vi "Shell and Tube Heat Exchanger 2.vi"() -> ()   [LabVIEW 2017]
uses:
  FlowSet S&THx.vi
  Level Set S&THx.vi
  Steam Set S&THx.vi
  Halt S&THx.vi
  <vilib>/addons/control/pid/pid.llb/PID Control Input Filter (DBL).vi
  <vilib>/addons/control/pid/pid.llb/PID Advanced (DBL).vi
  Flow Out S&THx.vi
  Level Out S&THx.vi
  Steam Out S&THx.vi
  <vilib>/addons/control/pid/NI_PID_pid.lvlib
panel:
  in  "Recording Increment (sec)":dbl=0.3 min=0.1 max=100.0 step=0.1 format="%#_13g"
  in  "stop":bool
  out "Last Time Write":dbl format="%#_13g"
  in  "Replace File":bool
  in  "Enable 6":bool
  in  "error in (no error)":errorcluster
  out "Makeup Flowrate":dbl caption="L/min"
  out "Makeup Temperature":dbl caption="C"
  in  "Pump Switch":bool
  out "Water Inlet Temperature":dbl=22.229346791369398 format="%.1f"
  out "Water Outlet Temperature":dbl=22.816489944987293 format="%.1f"
  in  "Flowrate Setpoint (GPM)":dbl=40.0 min=0.0 max=50.0 format="%.2f"
  out "Water Flowrate":dbl=-0.0005338564515105265 format="%.2f"
  out "Flow Control Valve":dbl(slide)=100.0 scale=0.0..100.0
  in  "Manual Override (Flow)":bool=TRUE
  in  "Set Manual Valve Position (Flow)":dbl(slide)=100.0 scale=0.0..100.0
  in  "Level Setpoint (ft)":dbl=1.5 min=0.0 max=2.0 format="%.2f"
  out "Liquid Level in Tank":dbl=-0.5117058749718749 format="%.2f"
  out "Level Control Valve":dbl(slide)=0.045055175643920364 scale=0.0..100.0
  in  "Manual Override (Level)":bool=TRUE
  in  "Set Manual Valve Position (Level)":dbl(slide) scale=0.0..100.0
  in  "Kc (Flow)":dbl=0.74
  in  "Ti (Flow)":dbl=0.036 caption="(min)"
  in  "Td (Flow)":dbl caption="(min)"
  in  "Kc (Level)":dbl=-75.0
  in  "Ti (Level)":dbl=0.005 caption="(min)"
  in  "Td (Level)":dbl caption="(min)"
  out "House Steam Pressure":dbl=-37.74410859375 caption="psig" format="%#.6g"
  out "Tube-Side Pressure Drop":dbl=-3.6907662628125 caption="psig"
  in  "Main Power":bool
  in  "Steam Pressure Setpoint (psig)":dbl=10.0 min=0.0 max=45.0 format="%.2f"
  out "Steam Pressure":dbl=-38.330115825 caption="psig" format="%.2f"
  out "Steam Valve":dbl(slide) scale=0.0..100.0
  in  "Manual Control Override (Steam Pressure)":bool
  in  "Set Manual Valve Position (Steam Pressure)":dbl(slide) scale=0.0..100.0
  in  "Kc (Steam)":dbl=0.5
  in  "Ti (Steam)":dbl=0.05 caption="(min)"
  in  "Td (Steam)":dbl caption="(min)"
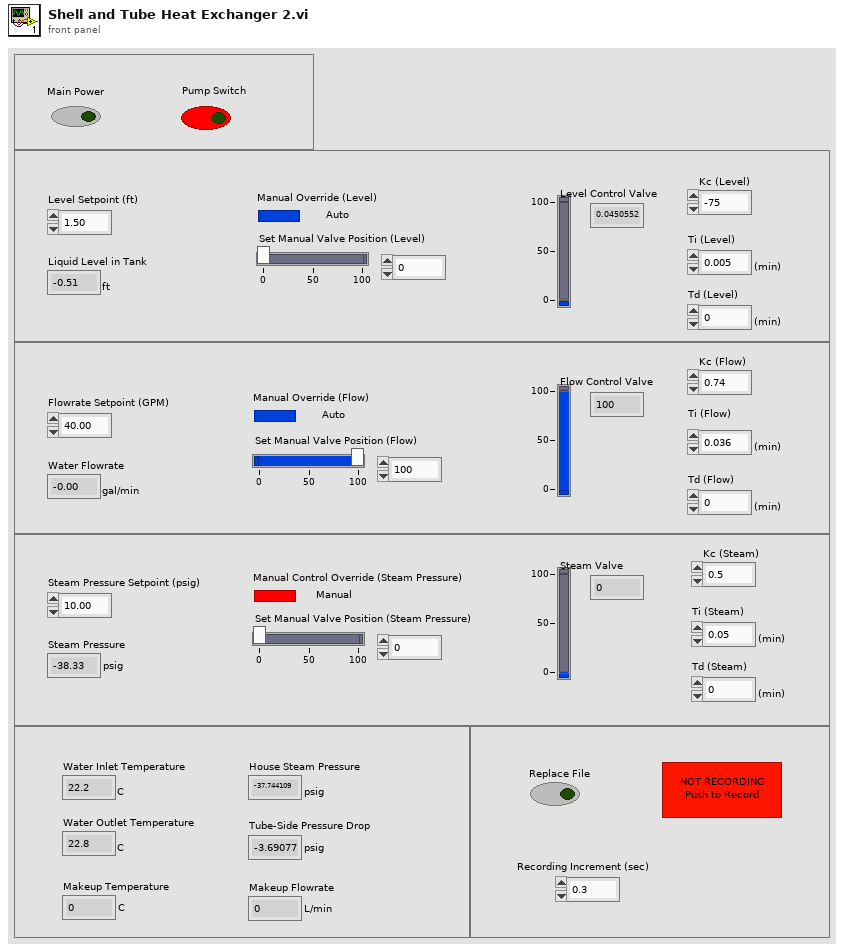
[diagram p1: front panel]
types:
  T1 = enum16{"open", "replace", "create", "open or create", "replace or create", "replace or create with confirmation"}
  T2 = cluster{"Kc (Flow)":dbl, "Ti (Flow)":dbl, "Td (Flow)":dbl}
  T3 = cluster{"Kc (Level)":dbl, "Ti (Level)":dbl, "Td (Level)":dbl}
  T4 = cluster{"Kc (Steam)":dbl, "Ti (Steam)":dbl, "Td (Steam)":dbl}
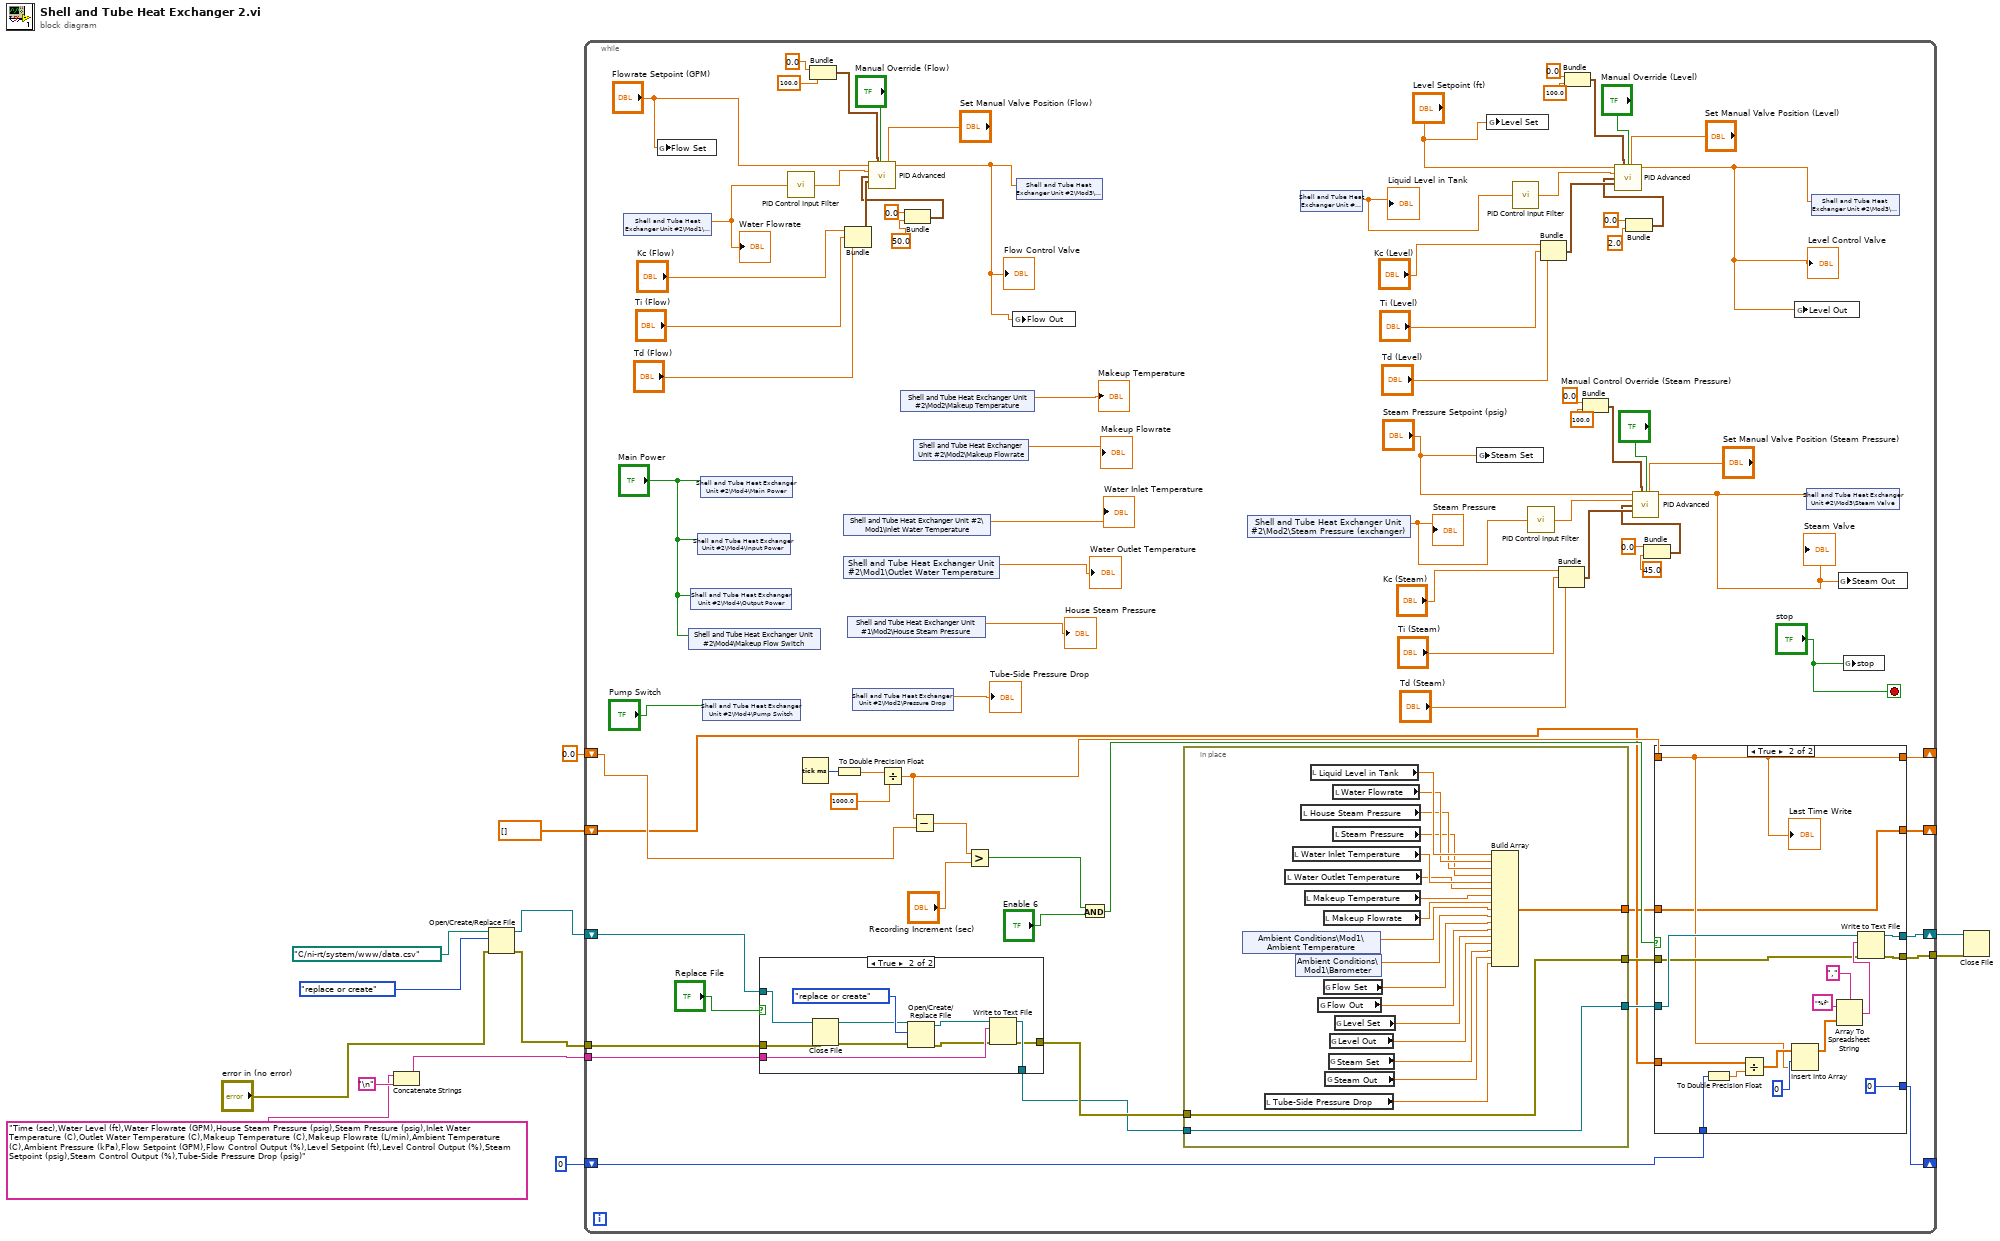
[diagram p0: block diagram]
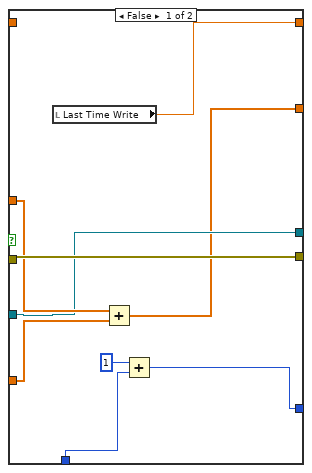
[diagram p2: hidden frame]
diagram:
  n1 = Concatenate Strings("Time (sec),Water Level (ft),Water Flowrate (GPM),House Steam Pressure (psig),Steam Pressure (psig),Inlet Water Temperature (C),Outlet Water Temperature (C),Makeup Temperature (C),Makeup Flowrate (L/min),Ambient Temperature (C),Ambient Pressure (kPa),Flow Setpoint (GPM),Flow Control Output (%),Level Setpoint (ft),Level Control Output (%),Steam Setpoint (psig),Steam Control Output (%),Tube-Side Pressure Drop (psig)", "\n") -> (w8:string)
  n2 = Open/Create/Replace File(file path (use dialog)=path "C:/ni-rt/system/www/data.csv" ("Filename"), error in="error in (no error)", operation (0:open)=T1."replace or create") -> (refnum out=w6:refnum<file>, error out=w7:errorcluster)  [unwired: 3 in, 1 out]
  n3 = while {
    tunnel: w8 -> [w25]
    tunnel: w7 -> [w33]
    shift-right: [w30] -> _
    shift-left: 0.0 ("Last Time Write") -> [w29]
    shift-right: [w28] -> w4
    shift-left: w6 -> [w27]
    tunnel: [w26] -> w5
    shift-right: [w16] -> _
    shift-left: dbl[] [] -> [w17]
    shift-right: [w14] -> _
    shift-left: 0 -> [w18]
    stop <- "stop" stop-if-true
    n4 = shared-variable "Shell and Tube Heat Exchanger Unit #2\\Mod1\\Water Flow"() -> (w47:dbl)  [unwired: 1 in, 1 out]
    "Water Flowrate" <- w47
    n5 = global write "FlowSet S&THx.vi" "Flow Set"("Flowrate Setpoint (GPM)") -> ()
    n6 = shared-variable "Shell and Tube Heat Exchanger Unit #2\\Mod4\\Makeup Flow Switch"("Main Power") -> ()  [unwired: 1 in, 1 out]
    n7 = shared-variable "Shell and Tube Heat Exchanger Unit #2\\Mod4\\Output Power"("Main Power") -> ()  [unwired: 1 in, 1 out]
    n8 = shared-variable "Shell and Tube Heat Exchanger Unit #2\\Mod4\\Input Power"("Main Power") -> ()  [unwired: 1 in, 1 out]
    n9 = shared-variable "Shell and Tube Heat Exchanger Unit #2\\Mod4\\Main Power"("Main Power") -> ()  [unwired: 1 in, 1 out]
    n10 = shared-variable "Shell and Tube Heat Exchanger Unit #2\\Mod4\\Pump Switch"("Pump Switch") -> ()  [unwired: 1 in, 1 out]
    n11 = case shown="True" "Replace File" {
      tunnel: [w142 w151] -> w19
      tunnel: w25 -> [_ w150]
      tunnel: w33 -> [w143 w147]
      tunnel: [w143 w148] -> w21
      tunnel: w27 -> [w142 w145]
      frame False {
      }
      frame True {
        n12 = Close File(refnum=w145, error in=w147) -> (path=w144:path, error out=w146:errorcluster)
        n13 = Open/Create/Replace File(file path (use dialog)=w144, error in=w146, operation (0:open)=T1."replace or create") -> (refnum out=w152:refnum<file>, error out=w149:errorcluster)  [unwired: 3 in, 1 out]
        n14 = Write to Text File(file (use dialog)=w152, text=w150, error in=w149) -> (refnum out=w151:refnum<file>, error out=w148:errorcluster)  [unwired: 1 in, 1 out]
      }
    }
    n15 = call-poly <vilib>:"PID Control Input Filter.vi"("input"=w47) -> ("output"=w46:dbl)  [unwired: 4 in]
    n16 = Tick Count (ms)() -> (millisecond timer value=w39:u32)
    n17 = Bundle(0.0, 100.0) -> (w73:cluster{dbl, dbl})  [unwired: 1 in]
    n18 = To Double Precision Float(number=w39) -> (double precision float=w37:dbl)
    n19 = shared-variable "Shell and Tube Heat Exchanger Unit #2\\Mod1\\Inlet Water Temperature"() -> (→"Water Inlet Temperature":dbl)  [unwired: 1 in, 1 out]
    n20 = shared-variable "Shell and Tube Heat Exchanger Unit #2\\Mod1\\Outlet Water Temperature"() -> (→"Water Outlet Temperature":dbl)  [unwired: 1 in, 1 out]
    n21 = Bundle("Kc (Flow)"="Kc (Flow)", "Ti (Flow)"="Ti (Flow)", "Td (Flow)"="Td (Flow)") -> (w92:T2)  [unwired: 1 in]
    n22 = shared-variable "Shell and Tube Heat Exchanger Unit #1\\Mod2\\House Steam Pressure"() -> (→"House Steam Pressure":dbl)  [unwired: 1 in, 1 out]
    n23 = shared-variable "Shell and Tube Heat Exchanger Unit #2\\Mod2\\Pressure Drop"() -> (→"Tube-Side Pressure Drop":dbl)  [unwired: 1 in, 1 out]
    n24 = Divide(x=w37, y=1000.0) -> (x/y=w31:dbl)
    n25 = shared-variable "Shell and Tube Heat Exchanger Unit #2\\Mod2\\Makeup Temperature"() -> (→"Makeup Temperature":dbl)  [unwired: 1 in, 1 out]
    n26 = Bundle(0.0, 50.0) -> (w70:cluster{dbl, dbl})  [unwired: 1 in]
    n27 = call-poly <vilib>:"PID Advanced.vi"("setpoint"="Flowrate Setpoint (GPM)", "output range"=w73, "auto? (T)"="Manual Override (Flow)", "manual control"="Set Manual Valve Position (Flow)", "process variable"=w46, "setpoint range"=w70, "PID gains"=w92) -> ("output"=w80:dbl)  [unwired: 7 in, 1 out]
    "Flow Control Valve" <- w80
    n28 = Subtract(x=w31, y=w29) -> (x-y=w35:dbl)
    n29 = shared-variable "Shell and Tube Heat Exchanger Unit #2\\Mod2\\Makeup Flowrate"() -> (→"Makeup Flowrate":dbl)  [unwired: 1 in, 1 out]
    n30 = Greater?(x=w35, y="Recording Increment (sec)") -> (0:w34:bool)
    n31 = global write "Flow Out S&THx.vi" "Flow Out"(w80) -> ()
    n32 = shared-variable "Shell and Tube Heat Exchanger Unit #2\\Mod3\\Flow Valve"(w80) -> ()  [unwired: 1 in, 1 out]
    n33 = And(x=w34, y="Enable 6") -> (x .and. y?=w32:bool)
    n34 = in-place {
      in-place-border: [w99] -> w22
      in-place-border: w21 -> [w99]
      in-place-border: [w98] -> w20
      in-place-border: w19 -> [w98]
      in-place-border: [w97] -> w15
      n35 = shared-variable "Ambient Conditions\\Mod1\\Ambient Temperature"() -> (w108:dbl)  [unwired: 1 in, 1 out]
      n36 = local read "Tube-Side Pressure Drop"() -> (w100:dbl)
      n37 = local read "Water Outlet Temperature"() -> (w111:dbl)
      n38 = local read "Water Inlet Temperature"() -> (w112:dbl)
      n39 = shared-variable "Ambient Conditions\\Mod1\\Barometer"() -> (w107:dbl)  [unwired: 1 in, 1 out]
      n40 = local read "House Steam Pressure"() -> (w114:dbl)
      n41 = local read "Makeup Temperature"() -> (w110:dbl)
      n42 = local read "Liquid Level in Tank"() -> (w116:dbl)
      n43 = global read "Flow Out S&THx.vi" "Flow Out"() -> (w105:dbl)
      n44 = local read "Makeup Flowrate"() -> (w109:dbl)
      n45 = global read "FlowSet S&THx.vi" "Flow Set"() -> (w106:dbl)
      n46 = global read "Steam Out S&THx.vi" "Steam Out"() -> (w101:dbl)
      n47 = global read "Steam Set S&THx.vi" "Steam Set"() -> (w102:dbl)
      n48 = global read "Level Out S&THx.vi" "Level Out"() -> (w103:dbl)
      n49 = local read "Water Flowrate"() -> (w115:dbl)
      n50 = local read "Steam Pressure"() -> (w113:dbl)
      n51 = global read "Level Set S&THx.vi" "Level Set"() -> (w104:dbl)
      n52 = Build Array(w116, w115, w114, w113, w112, w111, w110, w109, w108, w107, w106, w105, w104, w103, w102, w101, w100) -> (w97:dbl[])
    }
    n53 = shared-variable "Shell and Tube Heat Exchanger Unit #2\\Mod2\\Steam Pressure (exchanger)"() -> (w45:dbl)  [unwired: 1 in, 1 out]
    "Steam Pressure" <- w45
    n54 = shared-variable "Shell and Tube Heat Exchanger Unit #2\\Mod2\\Level"() -> (w50:dbl)  [unwired: 1 in, 1 out]
    "Liquid Level in Tank" <- w50
    n55 = global write "Steam Set S&THx.vi" "Steam Set"("Steam Pressure Setpoint (psig)") -> ()
    n56 = global write "Level Set S&THx.vi" "Level Set"("Level Setpoint (ft)") -> ()
    n57 = call-poly <vilib>:"PID Control Input Filter.vi"("input"=w50) -> ("output"=w48:dbl)  [unwired: 4 in]
    n58 = call-poly <vilib>:"PID Control Input Filter.vi"("input"=w45) -> ("output"=w44:dbl)  [unwired: 4 in]
    n59 = Bundle("Kc (Level)"="Kc (Level)", "Ti (Level)"="Ti (Level)", "Td (Level)"="Td (Level)") -> (w94:T3)  [unwired: 1 in]
    n60 = Bundle("Kc (Steam)"="Kc (Steam)", "Ti (Steam)"="Ti (Steam)", "Td (Steam)"="Td (Steam)") -> (w63:T4)  [unwired: 1 in]
    n61 = Bundle(0.0, 100.0) -> (w76:cluster{dbl, dbl})  [unwired: 1 in]
    n62 = Bundle(0.0, 100.0) -> (w58:cluster{dbl, dbl})  [unwired: 1 in]
    n63 = Bundle(0.0, 2.0) -> (w67:cluster{dbl, dbl})  [unwired: 1 in]
    n64 = call-poly <vilib>:"PID Advanced.vi"("setpoint"="Level Setpoint (ft)", "output range"=w76, "auto? (T)"="Manual Override (Level)", "manual control"="Set Manual Valve Position (Level)", "process variable"=w48, "setpoint range"=w67, "PID gains"=w94) -> ("output"=w49:dbl)  [unwired: 7 in, 1 out]
    "Level Control Valve" <- w49
    n65 = Bundle(0.0, 45.0) -> (w55:cluster{dbl, dbl})  [unwired: 1 in]
    n66 = call-poly <vilib>:"PID Advanced.vi"("setpoint"="Steam Pressure Setpoint (psig)", "output range"=w58, "auto? (T)"="Manual Control Override (Steam Pressure)", "manual control"="Set Manual Valve Position (Steam Pressure)", "process variable"=w44, "setpoint range"=w55, "PID gains"=w63) -> ("output"=w53:dbl)  [unwired: 7 in, 1 out]
    "Steam Valve" <- w53
    n67 = case shown="True" w32 {
      tunnel: w22 -> [w124 w135]
      tunnel: w20 -> [w118 w136]
      tunnel: w31 -> [_ w129]
      tunnel: [w125 w129] -> w30
      tunnel: [w118 w139] -> w28
      tunnel: [w124 w138] -> w26
      tunnel: w18 -> [w120 w131]
      tunnel: w17 -> [w122 w130]
      tunnel: [w117 w127] -> w16
      tunnel: w15 -> [w121 w127]
      tunnel: [w119 0 ("index")] -> w14
      frame False {
        n68 = local read "Last Time Write"() -> (w125:dbl)
        n69 = Add(x=w121, y=w122) -> (x+y=w117:dbl[])
        n70 = Add(x=1, y=w120) -> (x+y=w119:i32)
      }
      frame True {
        n71 = To Double Precision Float(number=w131) -> (double precision float=w134:dbl)
        n72 = Divide(x=w130, y=w134) -> (x/y=w133:dbl[])
        n73 = Insert Into Array(array=w133, index=0, new element=w129) -> (w128:dbl[])
        n74 = Array To Spreadsheet String(delimiter (Tab)=",", array=w128, 3:"%f" ("format string")) -> (spreadsheet string=w137:string)
        n75 = Write to Text File(file (use dialog)=w136, text=w137, error in=w135) -> (refnum out=w139:refnum<file>, error out=w138:errorcluster)  [unwired: 1 in, 1 out]
        "Last Time Write" <- w129
      }
    }
    n76 = global write "Level Out S&THx.vi" "Level Out"(w49) -> ()
    n77 = shared-variable "Shell and Tube Heat Exchanger Unit #2\\Mod3\\Steam Valve"(w53) -> ()  [unwired: 1 in, 1 out]
    n78 = shared-variable "Shell and Tube Heat Exchanger Unit #2\\Mod3\\Level Valve"(w49) -> ()  [unwired: 1 in, 1 out]
    n79 = global write "Steam Out S&THx.vi" "Steam Out"(w53) -> ()
    n80 = global write "Halt S&THx.vi" "stop"("stop") -> ()
  }
  n81 = Close File(refnum=w4, error in=w5) -> ()  [unwired: 2 out]
